vi "Periodic Tasks.vi"(8 "error in":errorcluster) -> ()   [LabVIEW 2014]
doc: "This VI runs in parallel to other tasks. It can contain as many user-defined periodic loops as you need. These can carry out PID or other sorts of timed response."
uses:
  <vilib>/Rock Robotics/WPI/Joystick/WPI_JoystickGetSetRefNum.vi
  <vilib>/Rock Robotics/WPI/RobotDrive/WPI_RobotDriveGetSetRefNum.vi
  Global Variables.vi
  <vilib>/addons/control/pid/pid.llb/PID (DBL).vi
  <vilib>/addons/control/pid/NI_PID_pid.lvlib
panel:
  in  "output range":cluster{"output high":dbl, "output low":dbl}={"output high"=100.0, "output low"=-100.0} {"output low" format="%.2f"; "output high" format="%.2f"}
  in  "PID gains 2":T1={"proportional gain (Kc)"=0.5, "integral time (Ti, min)"=0.0, "derivative time (Td, min)"=0.0} {"derivative time (Td, min)" format="%.3f"; "integral time (Ti, min)" format="%.3f"; "proportional gain (Kc)" format="%.3f"}
  in  "voltage (V)":dbl
  out "upper limit":dbl
  in  "PID gains":T1={"proportional gain (Kc)"=1.0, "integral time (Ti, min)"=0.01, "derivative time (Td, min)"=0.0} {"derivative time (Td, min)" format="%.3f"; "integral time (Ti, min)" format="%.3f"; "proportional gain (Kc)" format="%.3f"}
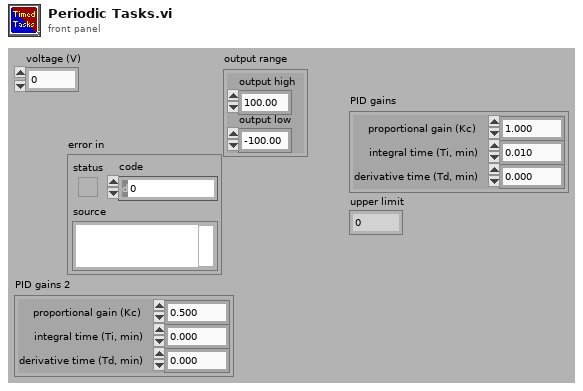
[diagram p1: front panel]
types:
  T1 = cluster{"proportional gain (Kc)":dbl, "integral time (Ti, min)":dbl, "derivative time (Td, min)":dbl}
  T2 = enum16{"Stop", "Three Tote", "Two Tote", "One Tote", "Step", "Top", "Home", "Joystick"}
  T3 = typedef "WPI_JoystickDevRef.ctl" = cluster{"Device":T4}
  T4 = typedef "WPI_JoystickDeviceEnum.ctl" = enum16{"USB 0", "USB 1", "USB 2", "USB 3", "USB 4", "USB 5"}
  T5 = typedef "WPI_RobotDriveDevRef.ctl" = cluster{"DevStatus":errorcluster, "Motors[]":T6[], "Square Inputs":bool, "Max Output":dbl}
  T6 = typedef "WPI_MotorControlDeviceRef.ctl" = cluster{"DeviceStatus":errorcluster, "Type":T7, "PWM":cluster{"Controller":T8, "PWM Channel":T9, "DeadBand":T10}, "CAN":cluster{"Device Number":u8, "Control Mode":T11, "Semaphore":T12, "Max Vout":dbl, "TalonSRX Control Mode":T13}, "Invert":bool, "TransformRef":T14, "InvTransformRef":T14}
  T7 = typedef "WPI_MotorControlType.ctl" = enum16{"PWM", "CAN", "CANTalonSRX"}
  T8 = typedef "FPGA_TypedefDigitalModule.ctl" = enum16{"Controller 1"}
  T9 = typedef "FPGA_DIOPWMChannel.ctl" = enum8{"PWM 0", "PWM 1", "PWM 2", "PWM 3", "PWM 4", "PWM 5", "PWM 6", "PWM 7", "PWM 8", "PWM 9", "PWM MXP 0", "PWM MXP 1", "PWM MXP 2", "PWM MXP 3", "PWM MXP 4", "PWM MXP 5", "PWM MXP 6", "PWM MXP 7", "PWM MXP 8", "PWM MXP 9", "Invalid"}
  T10 = typedef "WPI_PWMDeadband.ctl" = cluster{"Name":string, "maxPositivePwm":i32, "minPositivePwm":i32, "centerPwm":i32, "maxNegativePwm":i32, "minNegativePwm":i32, "angularRange":u16}
  T11 = typedef "WPI_CANJaguar_ControlMode.ctl" = enum8{"Percent VBus", "Current", "Speed", "Position", "Voltage"}
  T12 = typedef "Semaphore RefNum" = refnum<k1>
  T13 = typedef "WPI_CANTalonSRX_APIControlMode.ctl" = enum8{"Percent VBus", "Speed", "Position", "Slave", "Unchanged / Invalid"}
  T14 = typedef "WPI_PWMTransform_ConPane.ctl" = refnum<vi>
  T15 = cluster{"JoystickDevRef":T3, "RobotDriveDevRef":T5}
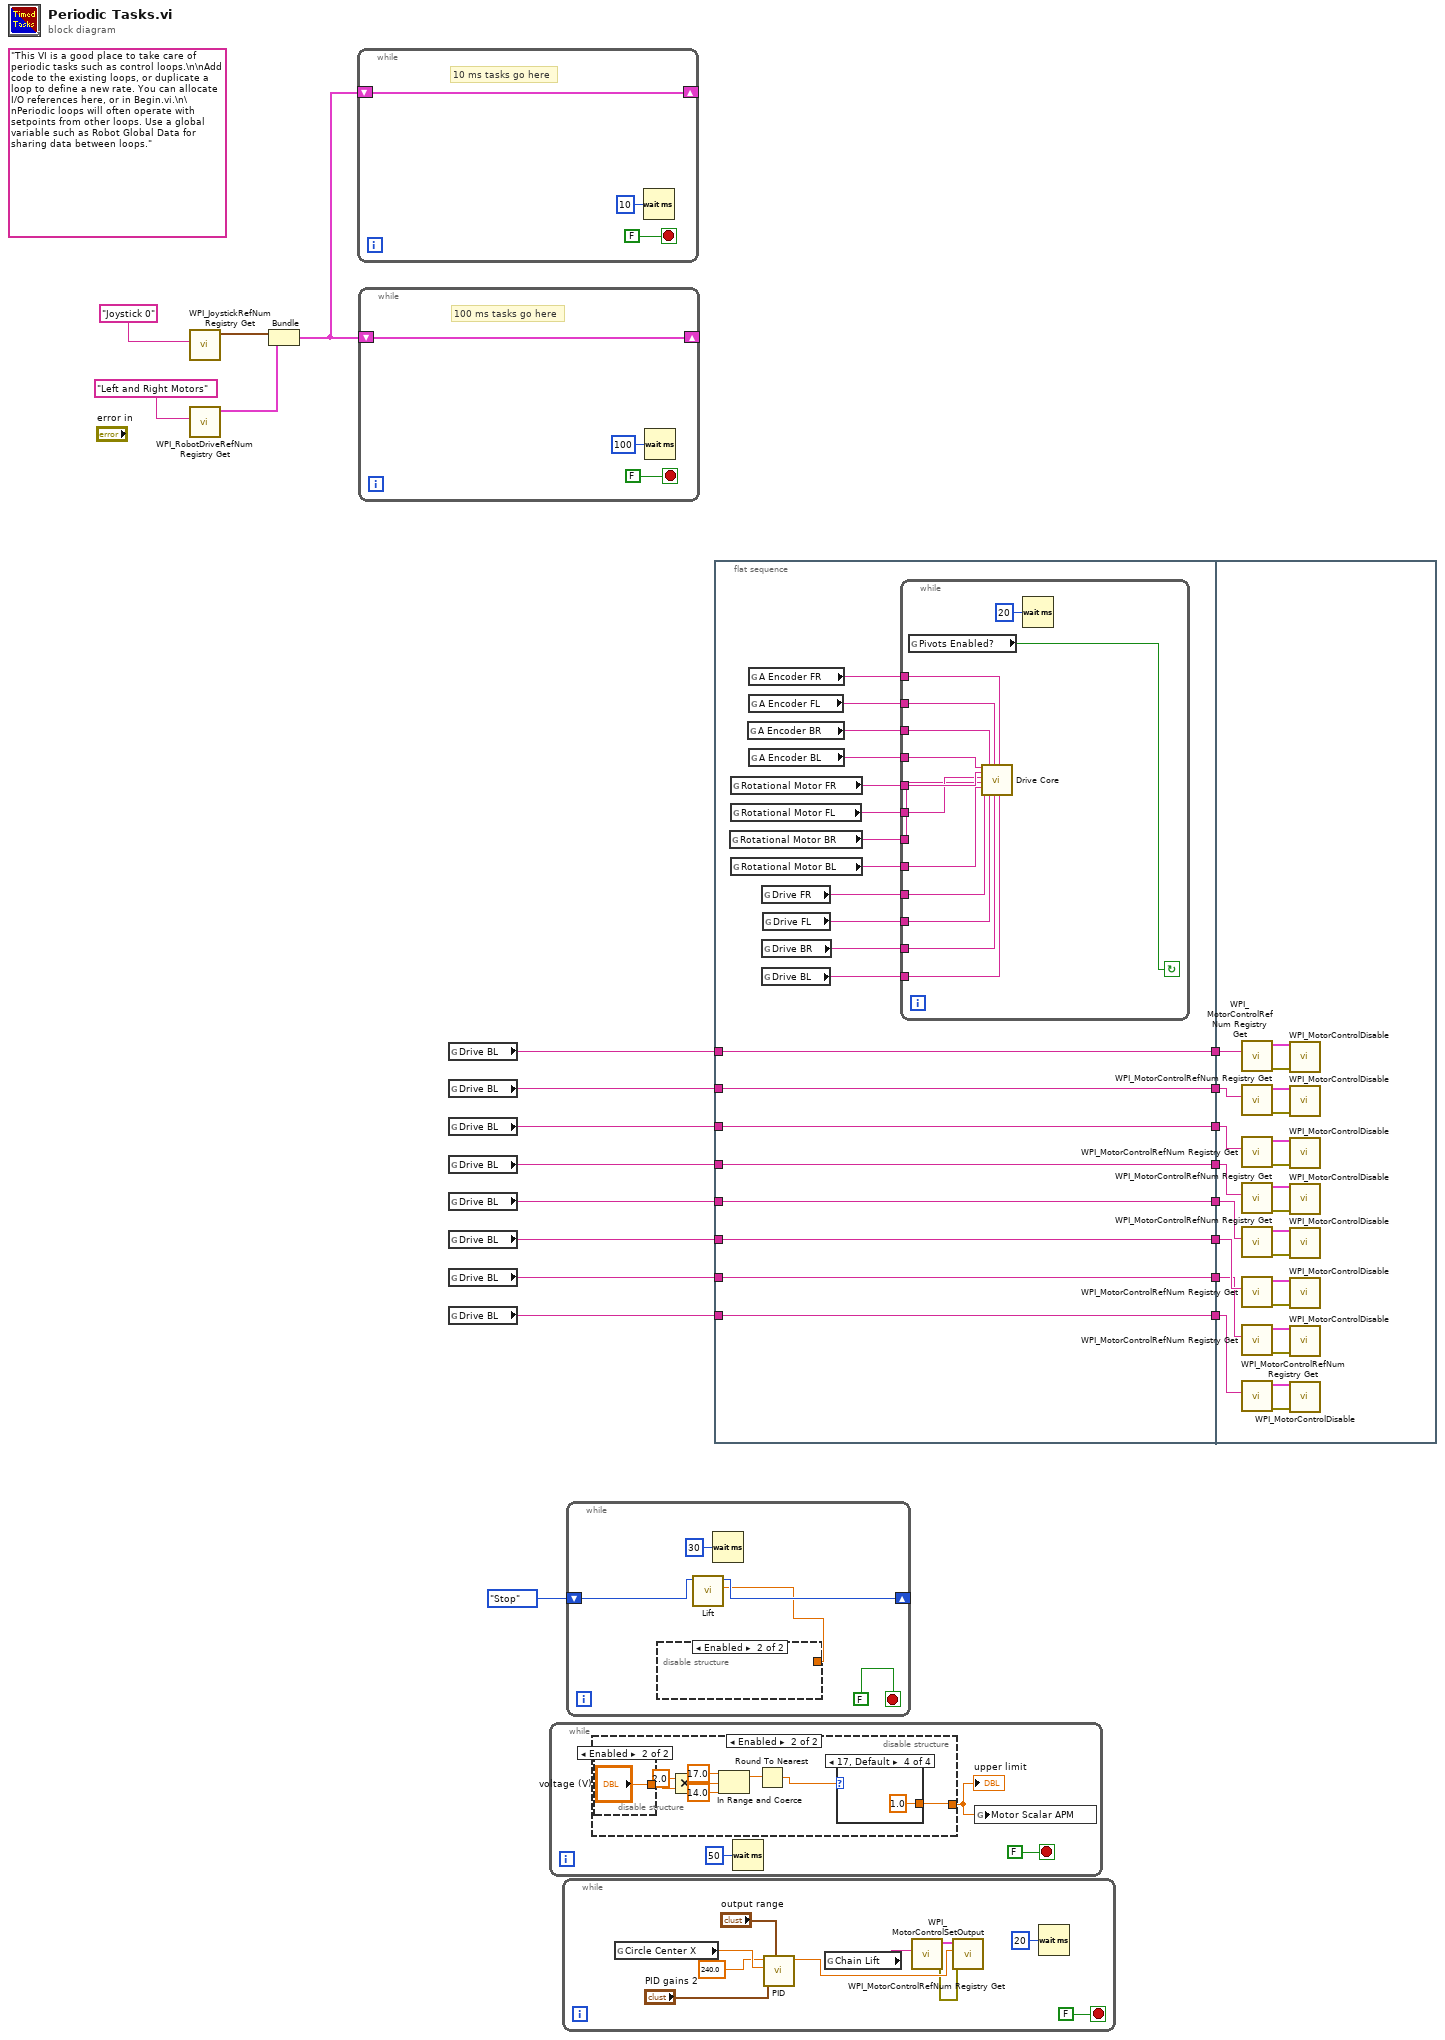
[diagram p0: block diagram]
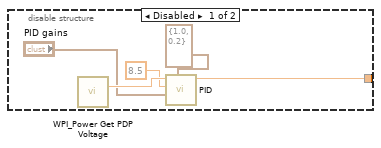
[diagram p2: hidden frame]
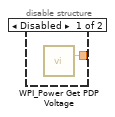
[diagram p3: hidden frame]
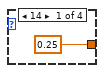
[diagram p4: hidden frame]
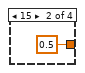
[diagram p5: hidden frame]
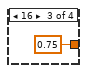
[diagram p6: hidden frame]
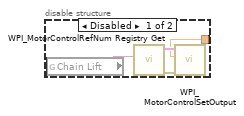
[diagram p7: hidden frame]
diagram:
  (unwired) "This VI is a good place to take care of periodic tasks such as control loops.\n\nAdd code to the existing loops, or duplicate a loop to define a new rate. You can allocate I/O references here, or in Begin.vi.\n\nPeriodic loops will often operate with setpoints from other loops. Use a global variable such as Robot Global Data for sharing data between loops."
  n1 = call <vilib>:"WPI_JoystickRefNum Registry Get.vi"("refnum name"="Joystick 0") -> ("JoystickDevRef"=w20:T3)  [unwired: 1 in, 9 out]
  n2 = call <vilib>:"WPI_RobotDriveRefNum Registry Get.vi"("refnum name"="Left and Right Motors") -> ("RobotDriveDevRef"=w19:T5)  [unwired: 1 in, 9 out]
  n3 = Bundle("JoystickDevRef"=w20, "RobotDriveDevRef"=w19) -> (w18:T15)  [unwired: 1 out]
  n4 = while {
    shift-right: [w23] -> _
    shift-left: w18 -> [w23]
    stop <- FALSE stop-if-true
    # "10 ms tasks go here"
    n5 = Wait (ms)(milliseconds to wait=u32 10) -> ()  [unwired: 1 out]
  }
  n6 = while {
    shift-right: [w26] -> _
    shift-left: w18 -> [w26]
    stop <- FALSE stop-if-true
    # "100 ms tasks go here"
    n7 = Wait (ms)(milliseconds to wait=u32 100) -> ()  [unwired: 1 out]
  }
  n8 = global read "Global Variables.vi" "Drive BL"() -> (w16:string)
  n9 = global read "Global Variables.vi" "Drive BL"() -> (w14:string)
  n10 = global read "Global Variables.vi" "Drive BL"() -> (w12:string)
  n11 = global read "Global Variables.vi" "Drive BL"() -> (w10:string)
  n12 = global read "Global Variables.vi" "Drive BL"() -> (w8:string)
  n13 = global read "Global Variables.vi" "Drive BL"() -> (w6:string)
  n14 = global read "Global Variables.vi" "Drive BL"() -> (w4:string)
  n15 = global read "Global Variables.vi" "Drive BL"() -> (w2:string)
  n16 = while {
    stop <- FALSE stop-if-true
    n17 = disable-structure shown="Enabled" {
      disable-tunnel: [w32 w38] -> w29
      frame Disabled {
        n18 = call <vilib>:"WPI_Power Get PDP Voltage.vi"() -> ("voltage (V)"=w35:dbl)  [unwired: 14 in, 1 out]
        n19 = call-poly <vilib>:"PID.vi"("output range"=cluster{"output high":dbl, "output low":dbl} {"output high"=1.0, "output low"=0.2}, "PID gains"="PID gains", "process variable"=8.5 ("setpoint"), "setpoint"=w35) -> ("output"=w32:dbl)  [unwired: 6 in, 1 out]
      }
      frame Enabled {
        n20 = disable-structure shown="Enabled" {
          disable-tunnel: [w45 "voltage (V)"] -> w44
          frame Disabled {
            n21 = call <vilib>:"WPI_Power Get PDP Voltage.vi"() -> ("voltage (V)"=w45:dbl)  [unwired: 14 in, 1 out]
          }
          frame Enabled {
          }
        }
        n22 = Multiply(x=2.0, y=w44) -> (x*y=w42:dbl)
        n23 = In Range and Coerce(upper limit=17.0, x=w42, lower limit=14.0) -> (coerced(x)=w40:dbl)  [unwired: 1 out]
        n24 = Round To Nearest(number=w40) -> (nearest integer value=w39:dbl)
        n25 = case shown="17, Default" w39 {
          tunnel: [0.25 ("upper limit") 0.5 ("upper limit") 0.75 ("upper limit") 1.0 ("upper limit")] -> w38
          frame 14 {
          }
          frame 15 {
          }
          frame 16 {
          }
          frame 17, Default {
          }
        }
      }
    }
    "upper limit" <- w29
    n26 = Wait (ms)(milliseconds to wait=u32 50) -> ()  [unwired: 1 out]
    n27 = global write "Global Variables.vi" "Motor Scalar APM"(w29) -> ()
  }
  n28 = while {
    stop <- FALSE stop-if-true
    n29 = global read "Global Variables.vi" "Circle Center X"() -> (w60:sgl)
    n30 = call-poly <vilib>:"PID.vi"("output range"="output range", "PID gains"="PID gains 2", "process variable"=w60, "setpoint"=240.0) -> ("output"=w55:dbl)  [unwired: 6 in, 1 out]
    n31 = global read "Global Variables.vi" "Chain Lift"() -> (w57:string)
    n32 = call <vilib>:"WPI_MotorControlRefNum Registry Get.vi"("refnum name"=w57) -> ("error out"=w52:errorcluster, "MotorControlDevRef"=w56:T6)  [unwired: 9 in]
    n33 = call <vilib>:"WPI_MotorControlSetOutput.vi"("error in (no error)"=w52, "Output"=w55, "MotorControlDevRef"=w56) -> ()  [unwired: 6 in, 3 out]
    n34 = Wait (ms)(milliseconds to wait=u32 20) -> ()  [unwired: 1 out]
  }
  n35 = while {
    shift-right: [w63] -> _
    shift-left: T2."Stop" ("State Out") -> [w64]
    stop <- FALSE stop-if-true
    n36 = call "Lift.vi"("State"=w64) -> ("Lift Motor(Global...)"=w61:dbl, "State Out"=w63:T2)  [unwired: 9 in]
    n37 = disable-structure shown="Enabled" {
      disable-tunnel: w61 -> [w67 _]
      frame Disabled {
        n38 = global read "Global Variables.vi" "Chain Lift"() -> (w66:string)
        n39 = call <vilib>:"WPI_MotorControlRefNum Registry Get.vi"("refnum name"=w66) -> ("error out"=w69:errorcluster, "MotorControlDevRef"=w68:T6)  [unwired: 9 in]
        n40 = call <vilib>:"WPI_MotorControlSetOutput.vi"("error in (no error)"=w69, "Output"=w67, "MotorControlDevRef"=w68) -> ()  [unwired: 6 in, 3 out]
      }
      frame Enabled {
      }
    }
    n41 = Wait (ms)(milliseconds to wait=u32 30) -> ()  [unwired: 1 out]
  }
  n42 = flat-sequence {
    tunnel: [w77] -> w17
    tunnel: w16 -> [w77]
    tunnel: [w76] -> w15
    tunnel: w14 -> [w76]
    tunnel: [w75] -> w13
    tunnel: w12 -> [w75]
    tunnel: [w74] -> w11
    tunnel: w10 -> [w74]
    tunnel: [w73] -> w9
    tunnel: w8 -> [w73]
    tunnel: [w72] -> w7
    tunnel: w6 -> [w72]
    tunnel: [w71] -> w5
    tunnel: w4 -> [w71]
    tunnel: [w70] -> w3
    tunnel: w2 -> [w70]
    tunnel: w17 -> [w111]
    tunnel: w15 -> [w110]
    tunnel: w13 -> [w109]
    tunnel: w11 -> [w108]
    tunnel: w9 -> [w107]
    tunnel: w7 -> [w106]
    tunnel: w5 -> [w105]
    tunnel: w3 -> [w104]
    frame #0 {
      n43 = global read "Global Variables.vi" "Rotational Motor BR"() -> (w83:string)
      n44 = global read "Global Variables.vi" "Rotational Motor FR"() -> (w85:string)
      n45 = global read "Global Variables.vi" "Rotational Motor FL"() -> (w84:string)
      n46 = global read "Global Variables.vi" "Rotational Motor BL"() -> (w82:string)
      n47 = global read "Global Variables.vi" "A Encoder BR"() -> (w87:string)
      n48 = global read "Global Variables.vi" "A Encoder FR"() -> (w89:string)
      n49 = global read "Global Variables.vi" "A Encoder FL"() -> (w88:string)
      n50 = global read "Global Variables.vi" "A Encoder BL"() -> (w86:string)
      n51 = global read "Global Variables.vi" "Drive FR"() -> (w81:string)
      n52 = global read "Global Variables.vi" "Drive BR"() -> (w79:string)
      n53 = global read "Global Variables.vi" "Drive BL"() -> (w78:string)
      n54 = global read "Global Variables.vi" "Drive FL"() -> (w80:string)
      n55 = while {
        tunnel: w89 -> [w102]
        tunnel: w88 -> [w101]
        tunnel: w87 -> [w100]
        tunnel: w86 -> [w99]
        tunnel: w85 -> [w98]
        tunnel: w84 -> [w97]
        tunnel: w83 -> [w96]
        tunnel: w82 -> [w95]
        tunnel: w81 -> [w94]
        tunnel: w80 -> [w93]
        tunnel: w79 -> [w92]
        tunnel: w78 -> [w91]
        stop <- w103 continue-if-true
        n56 = global read "Global Variables.vi" "Pivots Enabled?"() -> (w103:bool)
        n57 = call "Drive Core.vi"("A Encoder BL"=w99, "Rotational Motor FR"=w98, "Rotational Motor FL"=w97, "Rotational Motor BR"=w96, "Rotational Motor BL"=w95, "Drive Motor FR"=w94, "A Encoder BR"=w100, "Drive Motor FL"=w93, "A Encoder FL"=w101, "Drive Motor BR"=w92, "A Encoder FR"=w102, "Drive Motor BL"=w91) -> ()  [unwired: 8 in]
        n58 = Wait (ms)(milliseconds to wait=u32 20) -> ()  [unwired: 1 out]
      }
    }
    frame #1 {
      n59 = call <vilib>:"WPI_MotorControlRefNum Registry Get.vi"("refnum name"=w111) -> ("error out"=w127:errorcluster, "MotorControlDevRef"=w126:T6)  [unwired: 9 in]
      n60 = call <vilib>:"WPI_MotorControlRefNum Registry Get.vi"("refnum name"=w110) -> ("error out"=w125:errorcluster, "MotorControlDevRef"=w124:T6)  [unwired: 9 in]
      n61 = call <vilib>:"WPI_MotorControlRefNum Registry Get.vi"("refnum name"=w109) -> ("error out"=w123:errorcluster, "MotorControlDevRef"=w122:T6)  [unwired: 9 in]
      n62 = call <vilib>:"WPI_MotorControlRefNum Registry Get.vi"("refnum name"=w108) -> ("error out"=w121:errorcluster, "MotorControlDevRef"=w120:T6)  [unwired: 9 in]
      n63 = call <vilib>:"WPI_MotorControlRefNum Registry Get.vi"("refnum name"=w107) -> ("error out"=w119:errorcluster, "MotorControlDevRef"=w118:T6)  [unwired: 9 in]
      n64 = call <vilib>:"WPI_MotorControlRefNum Registry Get.vi"("refnum name"=w106) -> ("error out"=w117:errorcluster, "MotorControlDevRef"=w116:T6)  [unwired: 9 in]
      n65 = call <vilib>:"WPI_MotorControlRefNum Registry Get.vi"("refnum name"=w105) -> ("error out"=w115:errorcluster, "MotorControlDevRef"=w114:T6)  [unwired: 9 in]
      n66 = call <vilib>:"WPI_MotorControlRefNum Registry Get.vi"("refnum name"=w104) -> ("error out"=w113:errorcluster, "MotorControlDevRef"=w112:T6)  [unwired: 9 in]
      n67 = call <vilib>:"WPI_MotorControlDisable.vi"("error in (no error)"=w127, "MotorControlDevRef"=w126) -> ()  [unwired: 8 in, 2 out]
      n68 = call <vilib>:"WPI_MotorControlDisable.vi"("error in (no error)"=w125, "MotorControlDevRef"=w124) -> ()  [unwired: 8 in, 2 out]
      n69 = call <vilib>:"WPI_MotorControlDisable.vi"("error in (no error)"=w123, "MotorControlDevRef"=w122) -> ()  [unwired: 8 in, 2 out]
      n70 = call <vilib>:"WPI_MotorControlDisable.vi"("error in (no error)"=w121, "MotorControlDevRef"=w120) -> ()  [unwired: 8 in, 2 out]
      n71 = call <vilib>:"WPI_MotorControlDisable.vi"("error in (no error)"=w119, "MotorControlDevRef"=w118) -> ()  [unwired: 8 in, 2 out]
      n72 = call <vilib>:"WPI_MotorControlDisable.vi"("error in (no error)"=w117, "MotorControlDevRef"=w116) -> ()  [unwired: 8 in, 2 out]
      n73 = call <vilib>:"WPI_MotorControlDisable.vi"("error in (no error)"=w115, "MotorControlDevRef"=w114) -> ()  [unwired: 8 in, 2 out]
      n74 = call <vilib>:"WPI_MotorControlDisable.vi"("error in (no error)"=w113, "MotorControlDevRef"=w112) -> ()  [unwired: 8 in, 2 out]
    }
  }
